vi "Find Workspace.vi"(8 "Error In":errorcluster, 10 "Control In":T2={"I-O.lvclass"=refnum, "Gantry"=refnum, "Dispenser"="COM1"}, 11 "Workspace In":refnum<class "Current Position.lvclass">) -> (0 "Error Out":errorcluster, 1 "Workspace Out":T1, 2 "Control Out":T2={"I-O.lvclass"=refnum, "Gantry"=refnum, "Dispenser"="COM1"}, 3 "Workspace Out":refnum<class "Current Position.lvclass">)   [LabVIEW 2018, in "Current Position.lvclass"]
uses:
  Current Position.lvclass
  Controller/Controllers.ctl
  Controller/I-O/I-O.lvclass
  C:/Program Files (x86)/Aerotech/A3200/LabVIEW/2010/Bin/Aerotech.A3200.dll
  Program Files (x86)/Aerotech/A3200/LabVIEW/2010/Bin/Aerotech.A3200.dll
  Workspace.ctl
  Controller/Motion/Motion.lvclass
  Controller/Controller.lvclass
  Fixture.lvclass
panel:
  in  "Workspace":T1
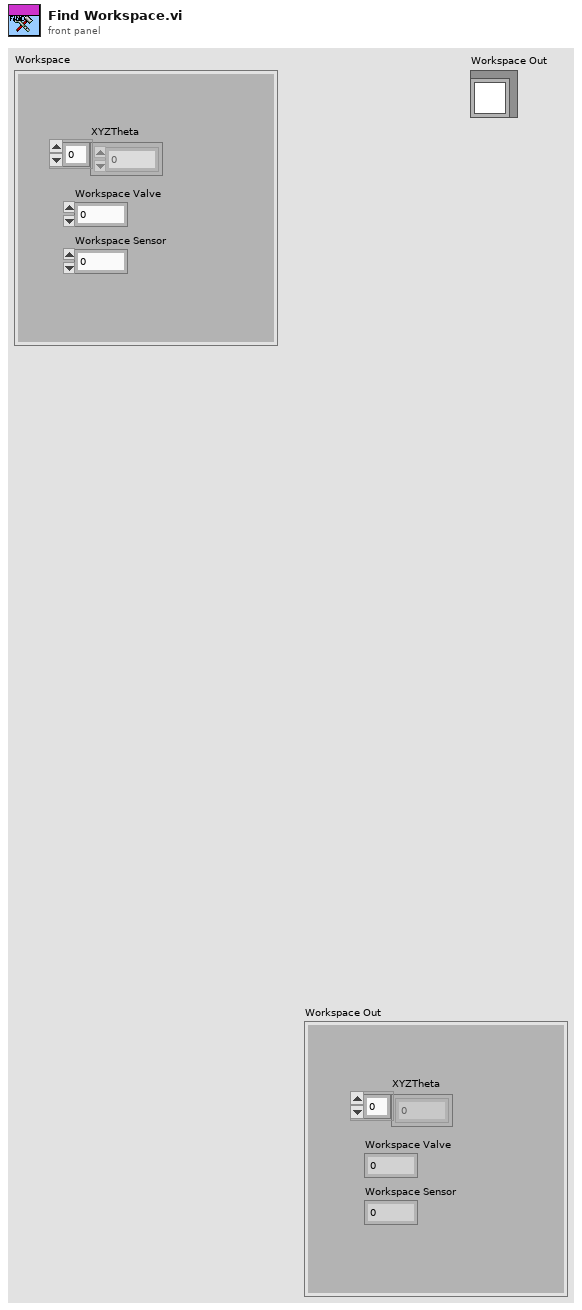
[diagram p1: front panel]
types:
  T1 = typedef "Fixture.lvclass/Workspace.ctl" = cluster{"XYZTheta":dbl[], "Workspace Valve":i32, "Workspace Sensor":i32}
  T2 = typedef "Controller.lvclass/Controllers.ctl" = cluster{"I-O.lvclass":refnum<class "I-O.lvclass">, "Gantry":refnum<k24>, "Dispenser":refnum<visa-resource-name>}
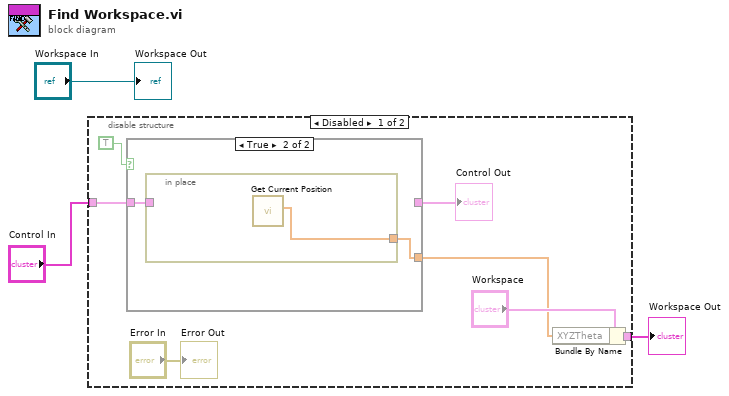
[diagram p0: block diagram]
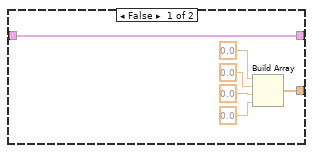
[diagram p2: hidden frame]
diagram:
  n1 = disable-structure shown="Disabled" {
    disable-tunnel: "Control In" -> [w10 _]
    disable-tunnel: [w6 _] -> w2
    frame Disabled {
      n2 = case shown="True" TRUE {
        tunnel: w10 -> [w16 w17]
        tunnel: [w16 _] -> w9
        tunnel: [w15 w18] -> w7
        frame False {
          n3 = Build Array(0.0, 0.0, 0.0, 0.0) -> (w15:dbl[])
        }
        frame True {
          n4 = in-place {
            in-place-border: [w19] -> w18
            in-place-border: w17 -> [_]
            n5 = call-dynamic "Get Current Position.vi"() -> ("XYZTheta Out"=w19:dbl[])  [unwired: 9 in, 2 out]
          }
        }
      }
      "Control Out" <- w9
      n6 = Bundle By Name(cluster="Workspace", "XYZTheta"=w7) -> (w6:T1)
      "Error Out" <- "Error In"
    }
    frame Enabled {
    }
  }
  "Workspace Out" <- w2
  "Workspace Out" <- "Workspace In"
